vi "SI prefix.vi"(1 "Numeric":dbl format="%#_6p") -> (0 "Answer":dbl)   [LabVIEW 2019, in "Instrument.DAQ.lvclass"]
uses:
  Instrument.DAQ.lvclass
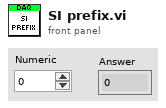
[diagram p1: front panel]
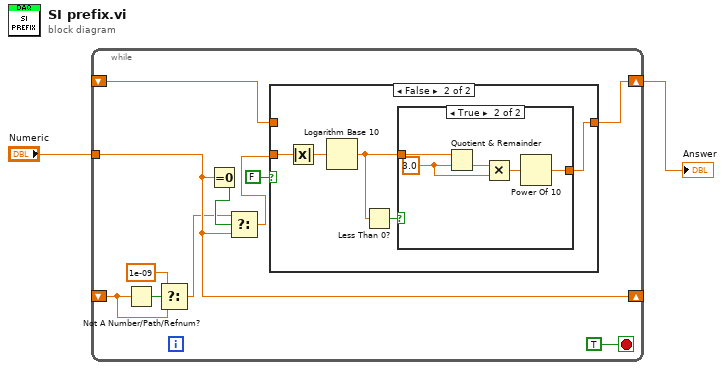
[diagram p0: block diagram]
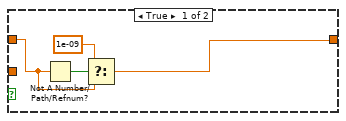
[diagram p2: hidden frame]
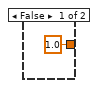
[diagram p3: hidden frame]
diagram:
  n1 = while {
    shift-right: [w13] -> w2
    shift-left: _ -> [w11]
    tunnel: "Numeric" -> [w8]
    shift-right: [w8] -> _
    shift-left: _ -> [w4]
    stop <- TRUE stop-if-true
    n2 = Not A Number/Path/Refnum?(number/path/refnum=w4) -> (NaN/Path/Refnum?=w6:bool)
    n3 = Select(t=1e-09, s=w6, f=w4) -> (s? t:f=w5:dbl)
    n4 = Equal To 0?(x=w8) -> (x = 0?=w9:bool)
    n5 = Select(t=w5, s=w9, f=w8) -> (s? t:f=w3:dbl)
    n6 = case shown="False" FALSE {
      tunnel: [w15 w22] -> w13
      tunnel: w3 -> [_ w18]
      tunnel: w11 -> [w14 _]
      frame True {
        n7 = Not A Number/Path/Refnum?(number/path/refnum=w14) -> (NaN/Path/Refnum?=w17:bool)
        n8 = Select(t=1e-09, s=w17, f=w14) -> (s? t:f=w15:dbl)
      }
      frame False {
        n9 = Absolute Value(x=w18) -> (abs(x)=w19:dbl)
        n10 = Logarithm Base 10(1:w19) -> (0:w21:dbl)
        n11 = Less Than 0?(x=w21) -> (x < 0?=w20:bool)
        n12 = case shown="True" w20 {
          tunnel: [1.0 w28] -> w22
          tunnel: w21 -> [_ w24]
          frame False {
          }
          frame True {
            w25 = 3.0 ("y")
            n13 = Quotient & Remainder(x=w24, y=w25) -> (floor(x/y)=w26:dbl)  [unwired: 1 out]
            n14 = Multiply(x=w26, y=w25) -> (x*y=w27:dbl)
            n15 = Power Of 10(x=w27) -> (10^x=w28:dbl)
          }
        }
      }
    }
  }
  "Answer" <- w2
